vi "Extract Nom Frequency.vi"(1 "String to Parse":string) -> (0 "Nominal Frequency":string)   [LabVIEW 2021]
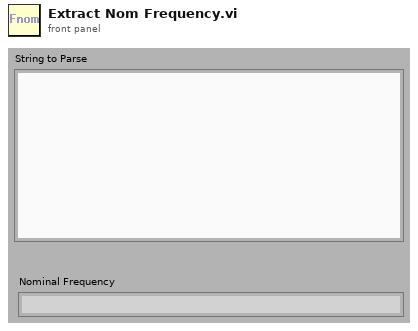
[diagram p1: front panel]
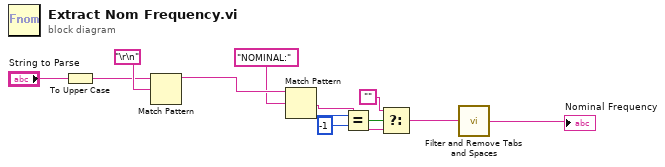
[diagram p0: block diagram]
diagram:
  n1 = To Upper Case(1:"String to Parse") -> (0:w9:string)
  n2 = Match Pattern(string=w9, regular expression="\r\n") -> (before substring=w11:string)  [unwired: 1 in, 3 out]
  n3 = Match Pattern(string=w11, regular expression="NOMINAL:") -> (after substring=w4:string, offset past match=w7:i32)  [unwired: 1 in, 2 out]
  n4 = Equal?(x=w7, y=-1) -> (x = y?=w5:bool)
  n5 = Select(t="", s=w5, f=w4) -> (s? t:f=w2:string)
  n6 = call "Filter and Remove Tabs and Spaces.vi"("Input String"=w2) -> ("Filtered String"=→"Nominal Frequency":string)
